vi "AT Set Int A.vi"(8 "error in (no error)":errorcluster, 9 "Value":i32, 10 "Feature":string, 11 "Handle":i32) -> (0 "error out":errorcluster, 3 "Status":i32)   [LabVIEW 2019]
doc: "Set Int\n\nOutput:\n I32 Status\n\n Input:\n I32 Handle\n String Feature\n I64 Handle\n\nThis function will modify the value of the specified feature, if the feature is of integer type. The function will return an error if the feature is read only or currently not writable or if the feature is either not an integer feature or is not implemented by the camera."
uses:
  atcoreA.dll
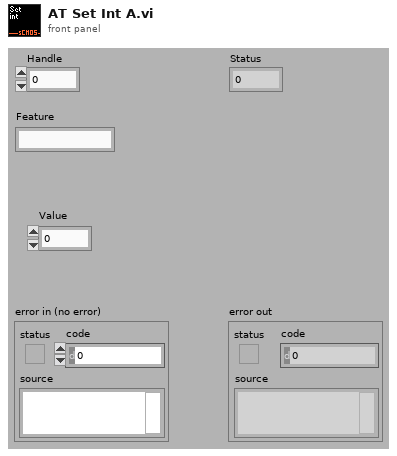
[diagram p1: front panel]
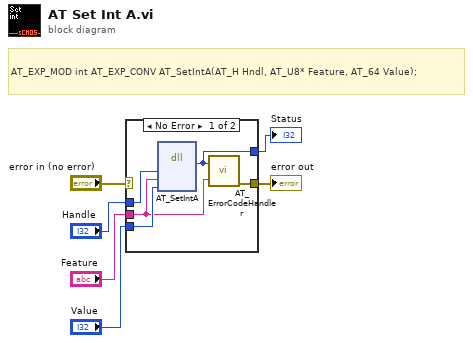
[diagram p0: block diagram]
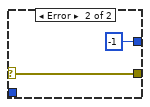
[diagram p2: hidden frame]
diagram:
  # "AT_EXP_MOD int AT_EXP_CONV AT_SetIntA(AT_H Hndl, AT_U8* Feature, AT_64 Value);"
  n1 = case shown="No Error" "error in (no error)" {
    selector: "error in (no error)" -> [_ w13]
    tunnel: [w8 -1 ("return type")] -> w6
    tunnel: "Handle" -> [w11 _]
    tunnel: "Feature" -> [w7 _]
    tunnel: "Value" -> [w10 _]
    tunnel: [w9 w13] -> w1
    frame No Error {
      n2 = dll-call lib="atcoreA.dll" fn="AT_SetIntA"("Handle"=w11, "Feature"=w7, "Value"=w10) -> ("Status"=w8:i32)  [unwired: 6 in, 2 out]
      n3 = call "AT_ErrorCodeHandler.vi"("Error"=w8, "Feature Name"=w7) -> ("error out"=w9:errorcluster)  [unwired: 5 in]
    }
    frame Error {
    }
  }
  "Status" <- w6
  "error out" <- w1
